vi "ParserPhysicalChannels.vi"(8 "error in (no error)":errorcluster, 10 "enums":T1[](array[typedef]), 11 "JSON item":string) -> (0 "error out":errorcluster, 2 "physical channels":T3[](array[typedef]), 3 "JSON item":string)   [LabVIEW 2018, in "Paser.lvlib"]
uses:
  Paser.lvlib
  Ctrl/PhysicalChannel.ctl
  Ctrl/Property.ctl
  Ctrl/Enum.ctl
  Ctrl/EnumValue.ctl
  9dd68465-a0ae-417f-8d6b-d89772fa241b.vi
  <vilib>/JDP Science/JSONtext/Find Item.vi
  <vilib>/JDP Science/JSONtext/String Subset.vi
  <vilib>/JDP Science/JSONtext/Parsing/Parse Full Path or Item Name.vi
  <vilib>/JDP Science/JSONtext/Offset/Find Item Locations by Path.vi
  <vilib>/JDP Science/JSONtext/JSON text to Variant.vi
  <vilib>/JDP Science/JSONtext/JSONtext.lvlib
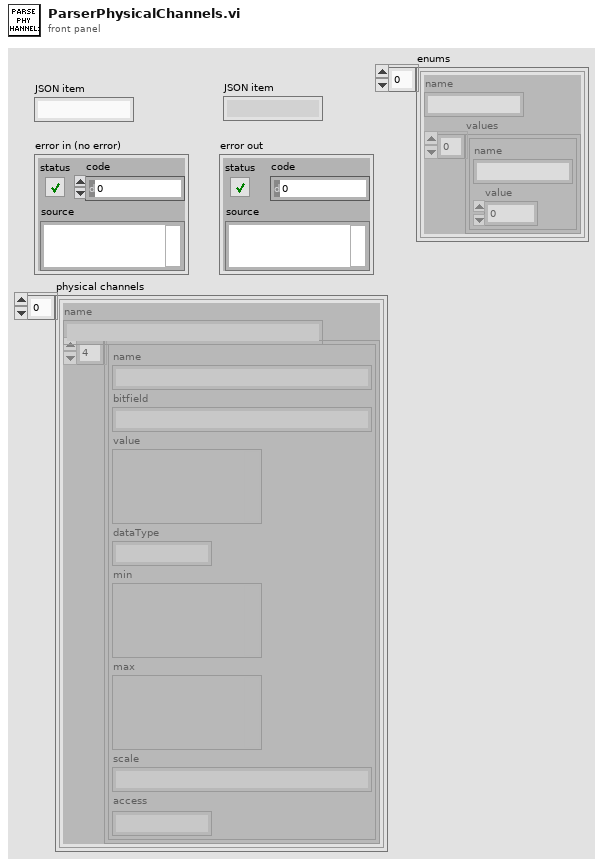
[diagram p1: front panel]
types:
  T1 = typedef "Enum.ctl" = cluster{"name":string, "values":T2[]}
  T2 = typedef "EnumValue.ctl" = cluster{"name":string, "value":i32}
  T3 = typedef "PhysicalChannel.ctl" = cluster{"name":string, "properties":T4[]}
  T4 = typedef "Property.ctl" = cluster{"name":string, "bitfield":string, "value":variant, "dataType":string, "min":variant, "max":variant, "scale":string, "access":string}
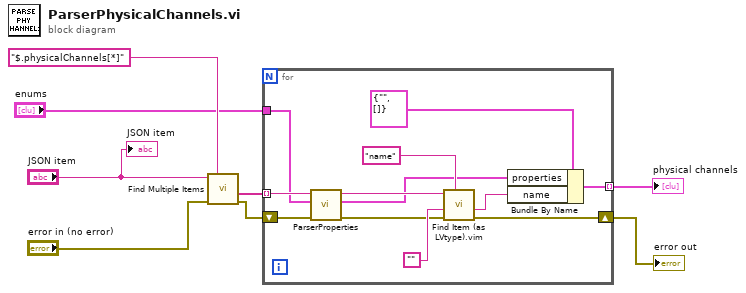
[diagram p0: block diagram]
diagram:
  n1 = call <vilib>:"Find Multiple Items.vi"("$Path or Item Name"="$.physicalChannels[*]", "error in (no error)"="error in (no error)", "JSON"="JSON item") -> ("error out"=w7:errorcluster, "<JSON>"=w5:string[])  [unwired: 5 in, 2 out]
  n2 = for {
    tunnel: w5 -> [w20] mode=indexing
    tunnel: [w17] -> w2 mode=indexing
    shift-right: [w13] -> w8
    shift-left: w7 -> [w15]
    tunnel: "enums" -> [w9]
    n3 = call "ParserProperties.vi"("error in (no error)"=w15, "enums"=w9, "JSON item"=w20) -> ("error out"=w14:errorcluster, "properties"=w11:T4[], "JSON item"=w12:string)  [unwired: 4 in]
    n4 = call "Find Item (as LVtype).vim"("$Path or Item Name"="name", "error in (no error)"=w14, "Data Type and Default Value"="" ("$Path or Item Name"), "JSON"=w12) -> ("error out"=w13:errorcluster, "Data"=w10:string)  [unwired: 4 in, 2 out]
    n5 = Bundle By Name(cluster=T3 {"name"="", "properties"=[]} ("PhysicalChannel"), "properties"=w11, "name"=w10) -> (w17:T3)
  }
  "error out" <- w8
  "physical channels" <- w2
  "JSON item" <- "JSON item"
